vi "Enqueue.vi"   [LabVIEW 2019, in "Acquire Mouse.lvlib"]
doc: "Function to enqueue a Message in a Queue of other Module."
uses:
  Acquire Mouse.lvlib
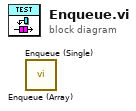
[diagram p0: block diagram]
diagram:
  n1 = call "Enqueue (Array).vi"() -> ()  [unwired: 10 in, 2 out]
  n2 = call "Enqueue (Single).vi"() -> ()  [unwired: 10 in, 2 out]
